vi "Processing Step.vi"(8 "error in (no error)":errorcluster, 11 "Controller in":refnum<class "Controller.lvclass">) -> (0 "error out":errorcluster, 2 "Array":T1[](array[typedef]), 3 "Controller out":refnum<class "Controller.lvclass">)   [LabVIEW 2020, in "HTTP Server.lvlib" / "Controller.lvclass"]
uses:
  Controller.lvclass
  Processing Step.ctl
  HTTP Server.lvlib
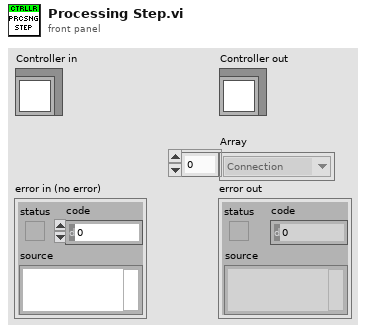
[diagram p1: front panel]
types:
  T1 = typedef "HTTP Server.lvlib/Processing Step.ctl" = enum16{"Connection", "Request", "Routing", "Controller Init", "Controller", "Response", "Cleanup", "Exception"}
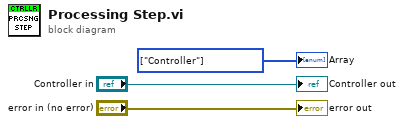
[diagram p0: block diagram]
diagram:
  w1 = T1[] [enum."Controller"] items=["Connection", "Request", "Routing", "Controller Init", "Controller", "Response", "Cleanup", "Exception"] ("Array")
  "error out" <- "error in (no error)"
  "Controller out" <- "Controller in"
  "Array" <- w1
